vi "SerialRead.vi"(0 "VISA resource name in":refnum<visa-resource-name>, 1 "错误输入（无错误）":errorcluster) -> (2 "VISA resource name out":refnum<visa-resource-name>, 3 "响应":string, 4 "错误输出":errorcluster)   [LabVIEW 2019]
panel:
  # "接收响应"
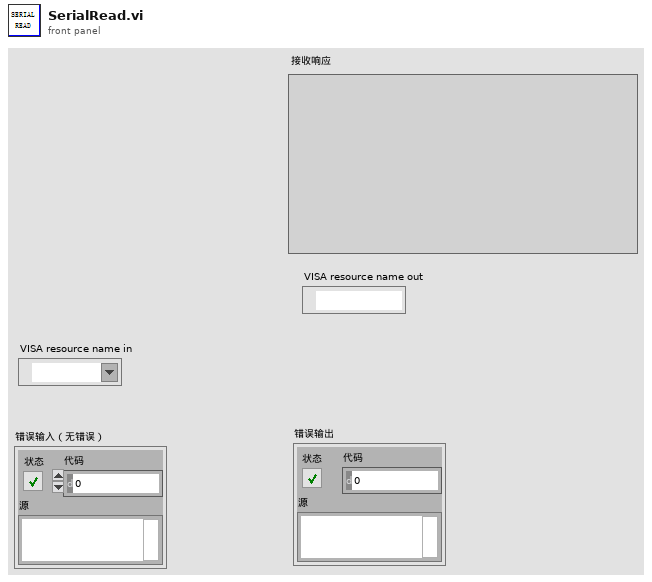
[diagram p1: front panel]
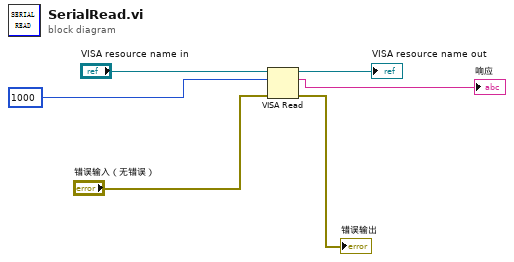
[diagram p0: block diagram]
diagram:
  n1 = VISA Read(VISA resource name="VISA resource name in", byte count=u32 1000 ("字节总数"), error in (no error)="错误输入（无错误）") -> (VISA resource name out=→"VISA resource name out":refnum<visa-resource-name>, read buffer=→"响应":string, error out=→"错误输出":errorcluster)  [unwired: 1 out]
